vi "Exercise 4-1.vi"(8 "error in (no error)":errorcluster, 9 "Min Temp":dbl, 10 "Max Temp":dbl, 11 "Current Temp":dbl) -> (0 "error out":errorcluster, 1 "Warning?":bool, 2 "Warning Text":string)   [LabVIEW 2014]
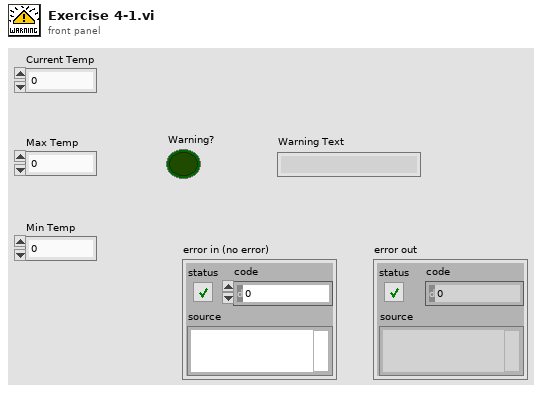
[diagram p1: front panel]
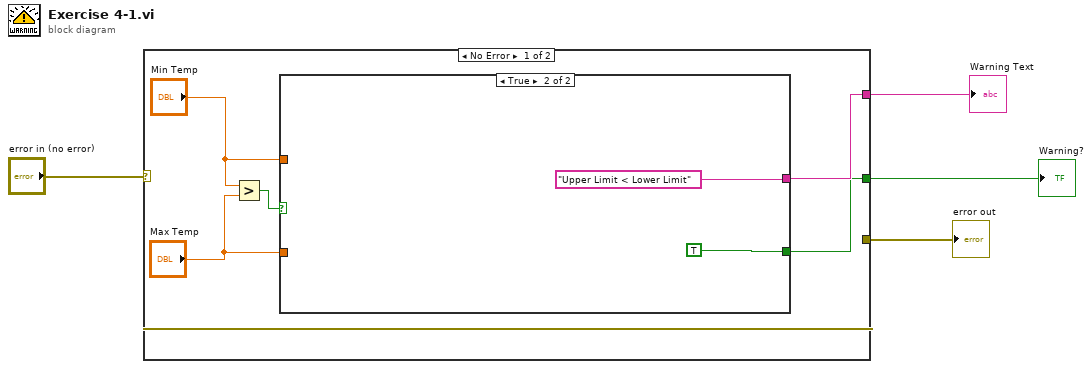
[diagram p0: block diagram]
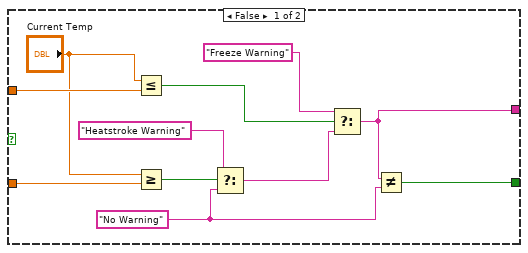
[diagram p2: hidden frame]
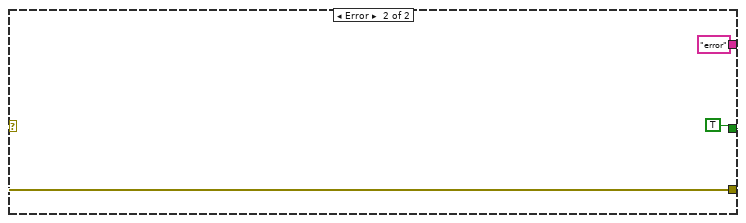
[diagram p3: hidden frame]
diagram:
  n1 = case shown="No Error" "error in (no error)" {
    selector: "error in (no error)" -> [w7 w26]
    tunnel: [w7 w26] -> w3
    tunnel: [w6 "error"] -> w2
    tunnel: [w5 TRUE] -> w1
    frame No Error {
      n2 = Greater?(x="Min Temp", y="Max Temp") -> (0:w10:bool)
      n3 = case shown="True" w10 {
        tunnel: "Min Temp" -> [w20 _]
        tunnel: "Max Temp" -> [w21 _]
        tunnel: [w14 "Upper Limit < Lower Limit"] -> w6
        tunnel: [w13 TRUE] -> w5
        frame False {
          w15 = "No Warning"
          n4 = Less Or Equal?(x="Current Temp", y=w20) -> (x <= y?=w18:bool)
          n5 = Greater Or Equal?(x="Current Temp", y=w21) -> (x >= y?=w16:bool)
          n6 = Select(t="Heatstroke Warning", s=w16, f=w15) -> (s? t:f=w12:string)
          n7 = Select(t="Freeze Warning", s=w18, f=w12) -> (s? t:f=w14:string)
          n8 = Not Equal?(x=w14, y=w15) -> (x != y?=w13:bool)
        }
        frame True {
        }
      }
    }
    frame Error {
    }
  }
  "error out" <- w3
  "Warning Text" <- w2
  "Warning?" <- w1
